vi "Create Channels.vi"(8 "error in (no error)":errorcluster, 10 "RSI Module in":refnum<class "9350.lvclass">, 11 "Parent Ref in":T1 format="%.0x") -> (0 "error out":errorcluster, 2 "RSI Module out":refnum<class "9350.lvclass">, 3 "Parent Ref out":T1 format="%.0x")   [LabVIEW 2017, in "Modules.lvlib" / "9350.lvclass"]
uses:
  9350.lvclass
  C:/Users/nitest/Documents/ni-official/niveristand-scan-engine-module-libraries/Source/RSI Module/RSI Module.lvclass
  <vilib>/NI Veristand/Custom Device API/Custom Device Item Ref.ctl
  <vilib>/NI Veristand/Custom Device API/Custom Device Channel Type.ctl
  <vilib>/NI Veristand/Custom Device API/Custom Device Channel.ctl
  RSI Module/Class Property Strings.vi
  RSI Module/Channel GUIDs.vi
  <vilib>/NI Veristand/Custom Device API/Custom Device API.lvlib
  RSI Module/RSI Module.lvclass
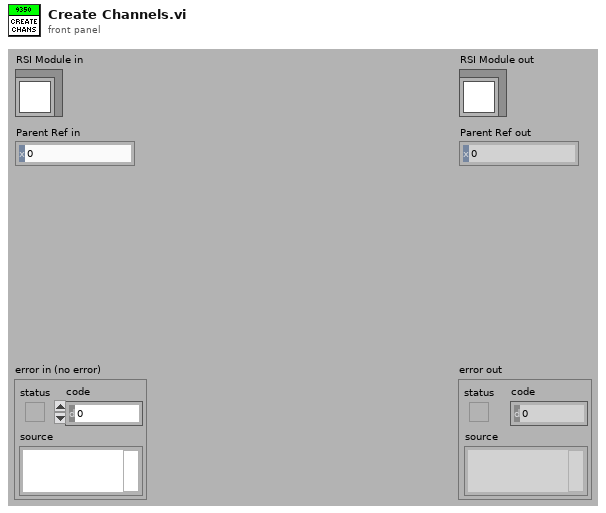
[diagram p1: front panel]
types:
  T1 = typedef "Custom Device API.lvlib/Custom Device Item Ref.ctl" = u64
  T2 = typedef "Custom Device API.lvlib/Custom Device Channel.ctl" = cluster{"Type":T3, "Units":string, "Default Value":dbl, "Faultable":bool, "Scalable":bool}
  T3 = typedef "Custom Device API.lvlib/Custom Device Channel Type.ctl" = enum16{"Input", "Output"}
  T4 = typedef "Modules.lvlib/RSI Module.lvclass/Channels.ctl" = cluster{"# Input Channels":i32, "# Output Channels":i32, "Channel Type":T5, "Units":string}
  T5 = typedef "Modules.lvlib/RSI Module.lvclass/Channel Type.ctl" = enum16{"Analog", "Digital"}
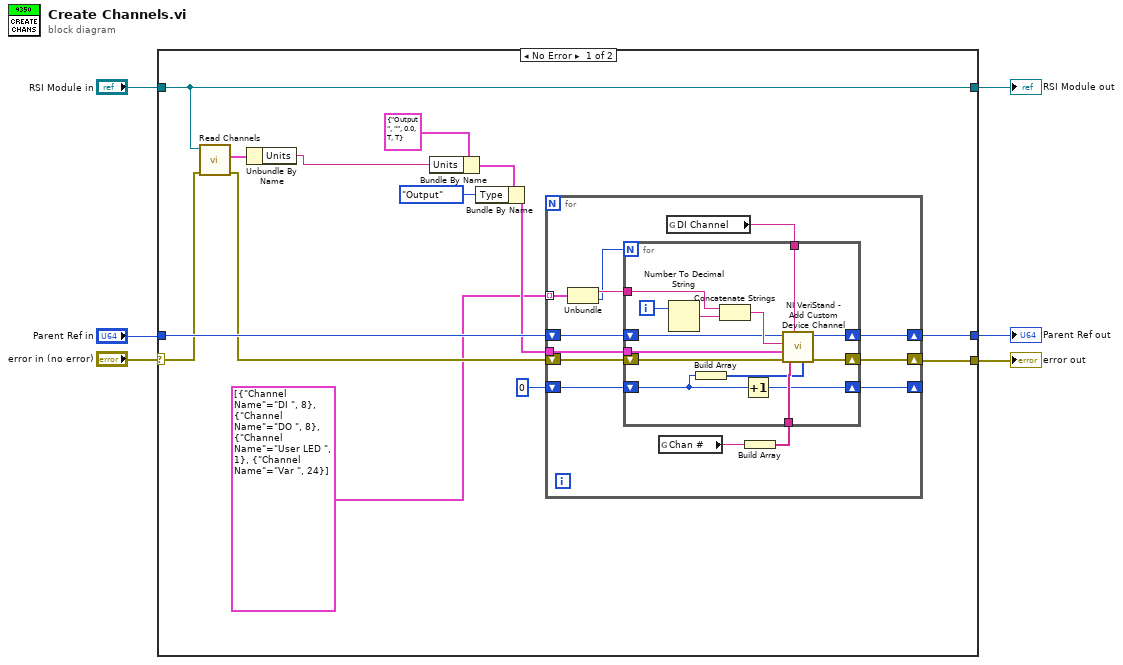
[diagram p0: block diagram]
diagram:
  n1 = case shown="No Error" "error in (no error)" {
    selector: "error in (no error)" -> [w18 w50]
    tunnel: [w7 w50] -> w5
    tunnel: [w15 w49] -> w3
    tunnel: "RSI Module in" -> [w15 w49]
    tunnel: "Parent Ref in" -> [w20 w48]
    tunnel: [w8 w48] -> w1
    frame No Error {
      n2 = call "Read Channels.vi"("error in (no error)"=w18, "RSI Module in"=w15) -> ("error out"=w17:errorcluster, "Channels"=w19:T4)  [unwired: 7 in, 1 out]
      n3 = Unbundle By Name(w19) -> ("Units"=w13:string)
      n4 = Bundle By Name(cluster=T2 {"Type"=enum."Output", "Units"="", "Default Value"=0.0, "Faultable"=TRUE, "Scalable"=TRUE} ("Channel"), "Units"=w13) -> (w11:T2)
      n5 = Bundle By Name(cluster=w11, "Type"=Custom_Device_Channel_Type."Output") -> (w16:T2)
      n6 = for {
        tunnel: w16 -> [w29]
        shift-right: [w26] -> w8
        shift-left: w20 -> [w33]
        shift-right: [w27] -> w7
        shift-left: w17 -> [w30]
        tunnel: cluster{"Channel Name":string, i32}[] [{"Channel Name"="DI ", 8}, {"Channel Name"="DO ", 8}, {"Channel Name"="User LED ", 1}, {"Channel Name"="Var ", 24}] -> [w25] mode=indexing
        shift-right: [w23] -> _
        shift-left: 0 -> [w22]
        n7 = Unbundle(w25) -> ("Channel Name"=w24:string, w21:i32)
        n8 = global read "Class Property Strings.vi" "Chan #"() -> (w32:string)
        n9 = global read "Channel GUIDs.vi" "DI Channel"() -> (w28:string)
        n10 = Build Array(w32) -> (w31:string[])
        n11 = for {
          N: w21 -> [_]
          tunnel: w24 -> [w45]
          tunnel: w29 -> [w37]
          tunnel: w28 -> [w38]
          tunnel: w31 -> [w42]
          shift-right: [w40] -> w27
          shift-left: w30 -> [w46]
          shift-right: [w39] -> w26
          shift-left: w33 -> [w43]
          shift-right: [w34] -> w23
          shift-left: w22 -> [w35]
          i -> [w36]
          n12 = Number To Decimal String(number=w36) -> (decimal integer string=w47:string)  [unwired: 1 in]
          n13 = Build Array(w35) -> (w41:i32[])
          n14 = Concatenate Strings(w45, w47) -> (w44:string)
          n15 = Increment(x=w35) -> (x+1=w34:i32)
          n16 = call <vilib>:"NI VeriStand - Add Custom Device Channel.vi"("Property Values"=w41, "Property names"=w42, "GUID (Default Channel)"=w38, "error in (no error)"=w46, "Channel"=w37, "Channel Name"=w44, "Parent Ref in"=w43) -> ("error out"=w40:errorcluster, "Parent Ref out"=w39:T1)  [unwired: 1 in, 2 out]
        }
      }
    }
    frame Error {
    }
  }
  "error out" <- w5
  "RSI Module out" <- w3
  "Parent Ref out" <- w1
